vi "RIO_AddToStack.vi"(1 "Number":string, 2 "Stack in":string[](array[string])) -> (0 "Stack out":string[](array[string]))   [LabVIEW 2012]
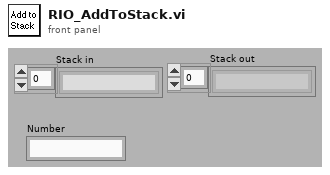
[diagram p1: front panel]
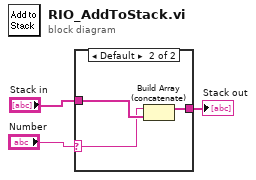
[diagram p0: block diagram]
diagram:
  n1 = case shown="Default" "Number" {
    selector: "Number" -> [_ w5]
    tunnel: "Stack in" -> [w4 w7]
    tunnel: [w4 w6] -> w2
    frame "" {
    }
    frame Default {
      n2 = Build Array (concatenate)(w5, w7) -> (w6:string[])
    }
  }
  "Stack out" <- w2
